vi "Check Configuration.vi"(8 "error in":errorcluster, 11 "framework configuration":T1) -> (0 "error out":errorcluster, 3 "framework configuration out":T1)   [LabVIEW 2017, in "DSF System Explorer.lvlib"]
uses:
  DSF System Explorer.lvlib
  DSF Core.lvlibp/Typedefs/DSF Engine Framework Configuration.ctl
  DSF Core.lvlibp/Typedefs/DSF Engine Plugin Configuration.ctl
  DSF Core.lvlibp/Typedefs/Core Plugin Configuration.ctl
  DSF Core.lvlibp/Typedefs/DSF Timing Info.ctl
  DSF Core.lvlibp/Typedefs/DSF Settings Info.ctl
  DSF Core.lvlibp/Typedefs/DSF Engine Plugin Thread Configuration.ctl
  DSF Core.lvlibp/Typedefs/Core Thread Configuration.ctl
  DSF Core.lvlibp/Typedefs/DSF Engine Transfer Group Configuration.ctl
  DSF Core.lvlibp/Typedefs/Core Group Configuration.ctl
  DSF Core.lvlibp/Typedefs/DSF Direction.ctl
  DSF Core.lvlibp/Typedefs/DSF Timeout Behavior.ctl
  DSF Core.lvlibp/Typedefs/DSF Engine Transfer Configuration.ctl
  DSF Core.lvlibp/Typedefs/Core Transfer Configuration.ctl
  DSF Core.lvlibp/Typedefs/DSF Engine Channel Configuration.ctl
  DSF Core.lvlibp/Typedefs/Core Channel Configuration.ctl
  DSF Core.lvlibp/Typedefs/DSF Data Type.ctl
  DSF Core.lvlibp
  DSF Core.lvlibp/Classes/Configuration/Core/Plugin/Plugin Configuration.lvclass
  DSF Core.lvlibp/Classes/Configuration/Core/Thread/Thread Configuration.lvclass
  DSF Core.lvlibp/Classes/Configuration/Core/Group/Group Configuration.lvclass
  DSF Core.lvlibp/Classes/Configuration/Core/Transfer/Transfer Configuration.lvclass
  DSF Core.lvlibp/Classes/Configuration/Core/Channel/Channel Configuration.lvclass
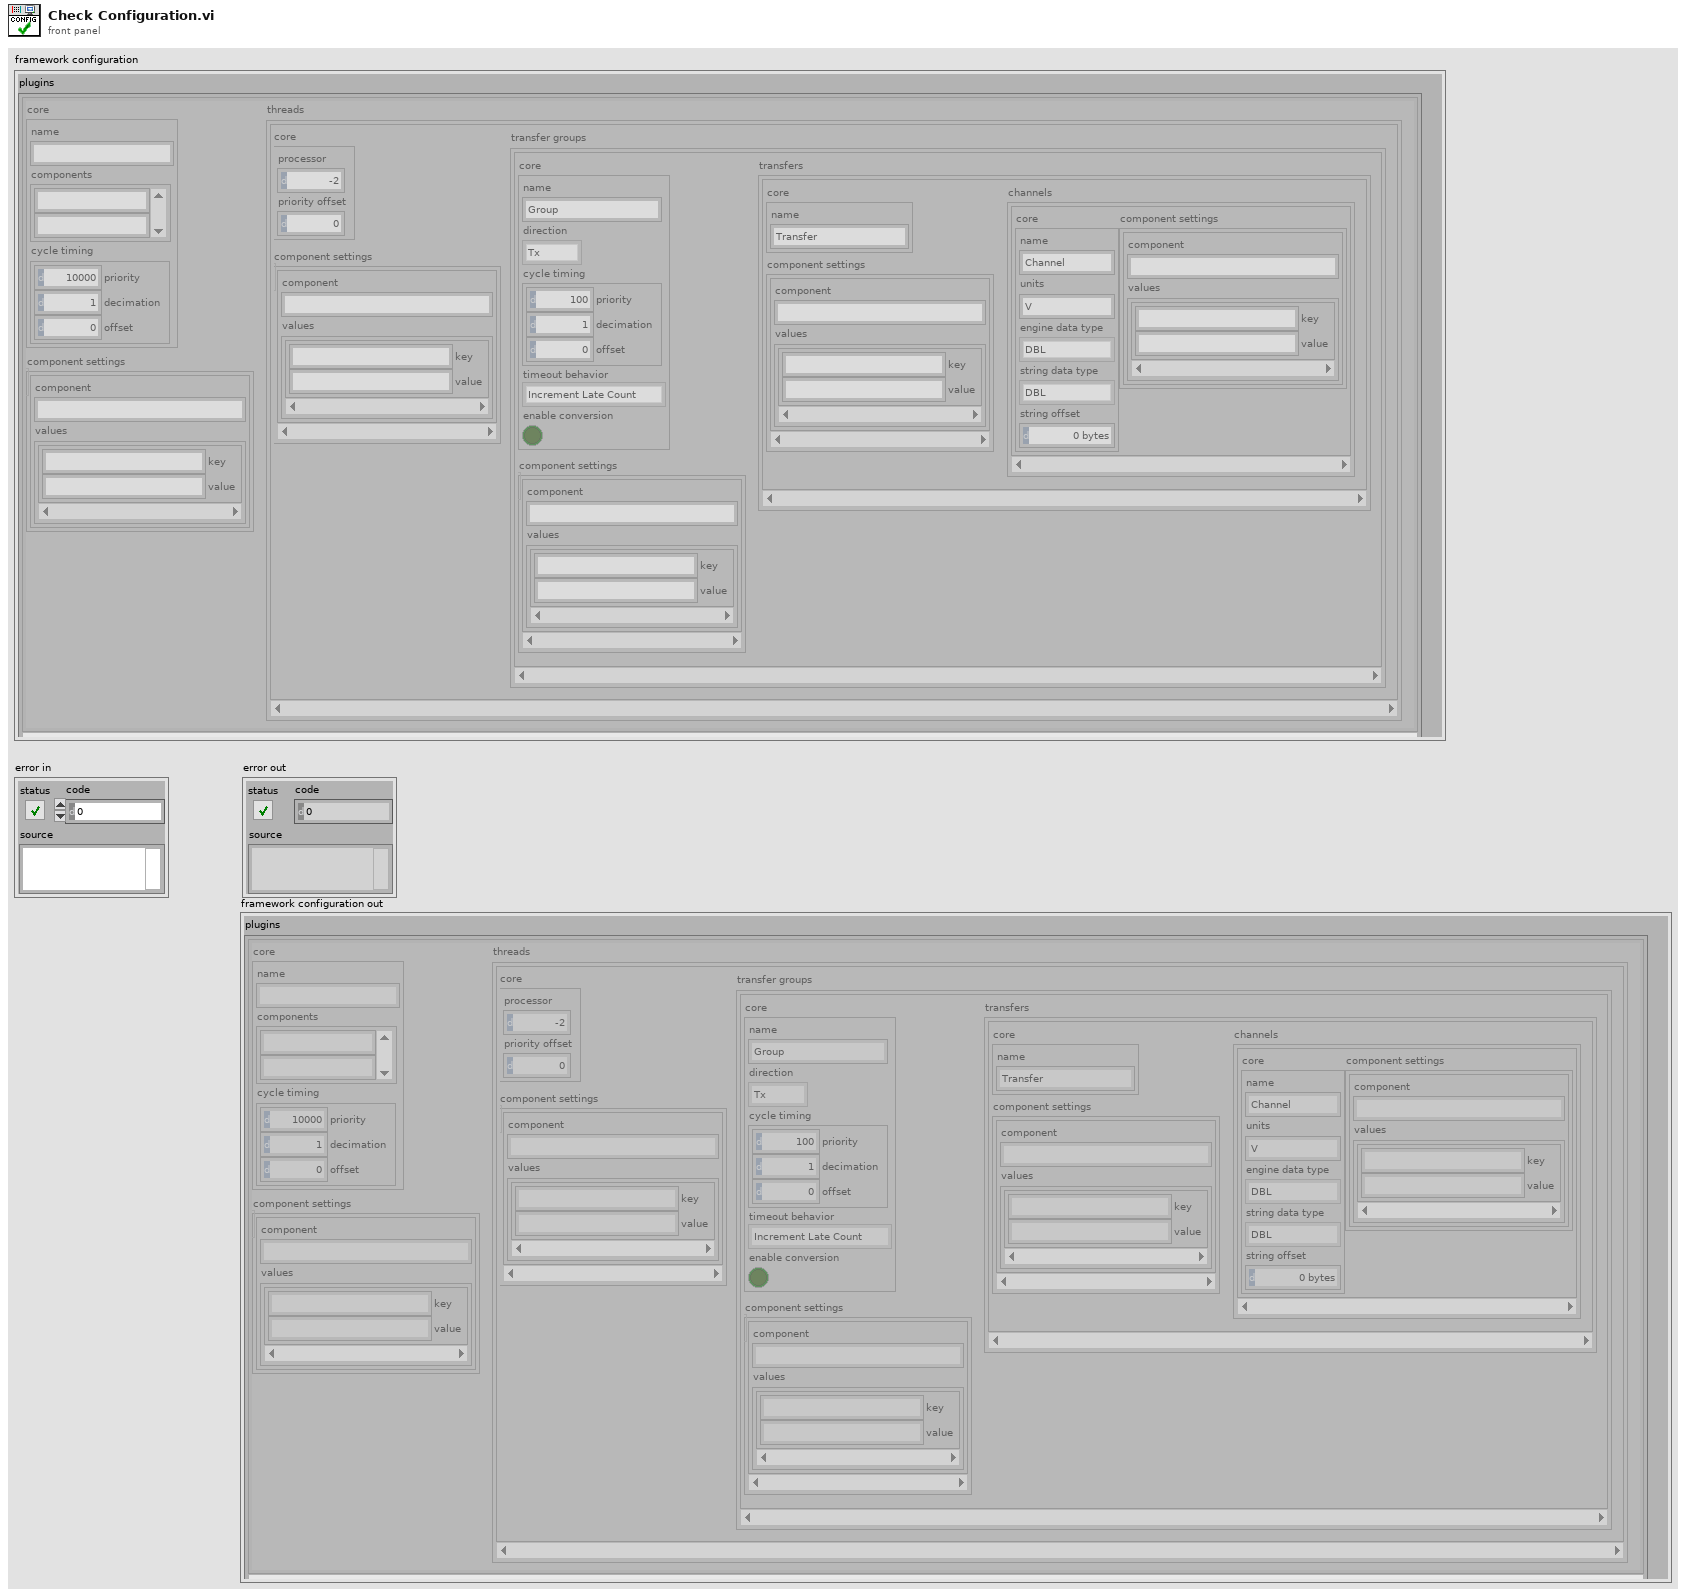
[diagram p1: front panel]
types:
  T1 = typedef "DSF Core.lvlibp/DSF Engine Framework Configuration.ctl" = cluster{"plugins":T2[]}
  T2 = typedef "DSF Core.lvlibp/DSF Engine Plugin Configuration.ctl" = cluster{"core":T3, "component settings":T5[], "threads":T6[]}
  T3 = typedef "DSF Core.lvlibp/Plugin Configuration.lvclass/Core Plugin Configuration.ctl" = cluster{"name":string, "components":string[], "cycle timing":T4}
  T4 = typedef "DSF Core.lvlibp/DSF Timing Info.ctl" = cluster{"priority":u64, "decimation":u64, "offset":u64}
  T5 = typedef "DSF Core.lvlibp/DSF Settings Info.ctl" = cluster{"component":string, "values":cluster{"key":string, "value":string}[]}
  T6 = typedef "DSF Core.lvlibp/DSF Engine Plugin Thread Configuration.ctl" = cluster{"core":T7, "component settings":T5[], "transfer groups":T8[]}
  T7 = typedef "DSF Core.lvlibp/Thread Configuration.lvclass/Core Thread Configuration.ctl" = cluster{"processor":i32, "priority offset":i16}
  T8 = typedef "DSF Core.lvlibp/DSF Engine Transfer Group Configuration.ctl" = cluster{"core":T9, "component settings":T5[], "transfers":T12[]}
  T9 = typedef "DSF Core.lvlibp/Group Configuration.lvclass/Core Group Configuration.ctl" = cluster{"name":string, "direction":T10, "cycle timing":T4, "timeout behavior":T11, "enable conversion":bool}
  T10 = typedef "DSF Core.lvlibp/DSF Direction.ctl" = enum8{"Tx", "Rx"}
  T11 = typedef "DSF Core.lvlibp/DSF Timeout Behavior.ctl" = enum8{"Increment Late Count", "Throw Error"}
  T12 = typedef "DSF Core.lvlibp/DSF Engine Transfer Configuration.ctl" = cluster{"core":T13, "component settings":T5[], "channels":T14[]}
  T13 = typedef "DSF Core.lvlibp/Transfer Configuration.lvclass/Core Transfer Configuration.ctl" = cluster{"name":string}
  T14 = typedef "DSF Core.lvlibp/DSF Engine Channel Configuration.ctl" = cluster{"core":T15, "component settings":T5[]}
  T15 = typedef "DSF Core.lvlibp/Channel Configuration.lvclass/Core Channel Configuration.ctl" = cluster{"name":string, "units":string, "engine data type":T16, "string data type":T16, "string offset":u64}
  T16 = typedef "DSF Core.lvlibp/DSF Data Type.ctl" = enum8{"Bool", "SGL", "DBL", "I8", "I16", "I32", "I64", "U8", "U16", "U32", "U64"}
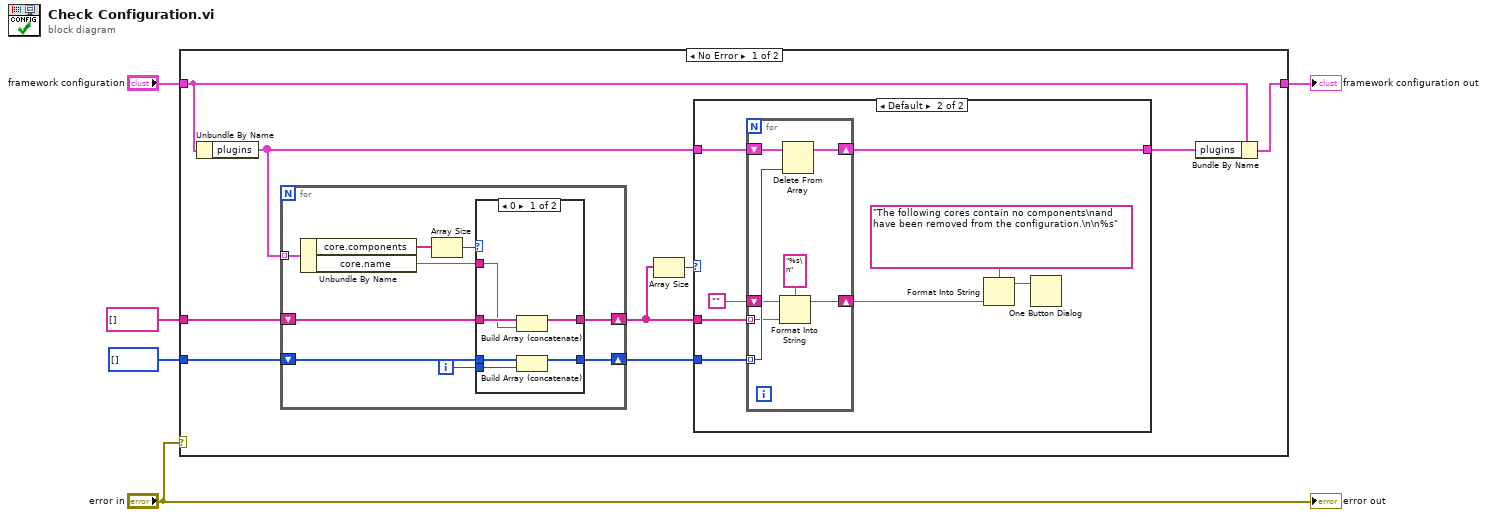
[diagram p0: block diagram]
diagram:
  n1 = case shown="No Error" "error in" {
    tunnel: "framework configuration" -> [w8 w48]
    tunnel: string[] [] -> [w14 _]
    tunnel: i32[] [] -> [w13 _]
    tunnel: [w6 w48] -> w2
    frame No Error {
      n2 = Unbundle By Name(w8) -> ("plugins"=w12:T2[])
      n3 = for {
        shift-right: [w31] -> w9
        shift-left: w14 -> [w36]
        tunnel: w12 -> [w35] mode=indexing
        shift-right: [w32] -> w11
        shift-left: w13 -> [w34]
        i -> [w33]
        n4 = Unbundle By Name(w35) -> ("core.components"=w38:string[], "core.name"=w37:string)
        n5 = Array Size(array=w38) -> (size(s)=w39:i32)
        n6 = case shown="0" w39 {
          tunnel: w37 -> [w44 _]
          tunnel: w36 -> [w45 w47]
          tunnel: [w43 w47] -> w31
          tunnel: w34 -> [w42 w46]
          tunnel: w33 -> [w41 _]
          tunnel: [w40 w46] -> w32
          frame 0 {
            n7 = Build Array (concatenate)(w45, w44) -> (w43:string[])
            n8 = Build Array (concatenate)(w42, w41) -> (w40:i32[])
          }
          frame Default {
          }
        }
      }
      n9 = Array Size(array=w9) -> (size(s)=w10:i32)
      n10 = case shown="Default" w10 {
        tunnel: w12 -> [w15 w23]
        tunnel: w11 -> [_ w22]
        tunnel: w9 -> [_ w21]
        tunnel: [w15 w16] -> w7
        frame 0 {
        }
        frame Default {
          n11 = for {
            shift-right: [w28] -> w16
            shift-left: w23 -> [w30]
            tunnel: w22 -> [w29] mode=indexing
            tunnel: w21 -> [w26] mode=indexing
            shift-right: [w24] -> w18
            shift-left: "" -> [w25]
            n12 = Format Into String(format string="%s\n", initial string=w25, w26) -> (resulting string=w24:string)  [unwired: 1 in, 1 out]
            n13 = Delete From Array(array=w30, index=w29) -> (array with subset deleted=w28:T2[])  [unwired: 1 in, 1 out]
          }
          n14 = Format Into String(format string="The following cores contain no components\nand have been removed from the configuration.\n\n%s", w18) -> (resulting string=w17:string)  [unwired: 2 in, 1 out]
          n15 = One Button Dialog(message=w17) -> ()  [unwired: 1 in, 1 out]
        }
      }
      n16 = Bundle By Name(cluster=w8, "plugins"=w7) -> (w6:T1)
    }
    frame Error {
    }
  }
  "framework configuration out" <- w2
  "error out" <- "error in"
